vi "climbStiltLoop.vi"() -> ()   [LabVIEW 2018]
uses:
  climbStiltStateEnum.ctl
  <vilib>/Platform/TimedLoop/XDataNode/timing_clust.ctl
  <vilib>/Platform/TimedLoop/XDataNode/nitl_modes.ctl
  <vilib>/Platform/TimedLoop/XDataNode/wakeup.ctl
  <vilib>/Rock Robotics/WPI/ThirdParty/Phoenix-LabVIEW/Motor Controller/Controls/CTRE_Phoenix_MotorControl_ControlMode.ctl
  climbPlatformEnum.ctl
  <vilib>/Rock Robotics/WPI/ThirdParty/Phoenix-LabVIEW/Motor Controller/Get/CTRE_Phoenix_MotorController_GetPulseWidthAll.vi
  <vilib>/addons/control/pid/pid.llb/PID (DBL).vi
  <vilib>/platform/TimedLoop/XDataNode/XDataNode.xnode
  <vilib>/addons/control/pid/NI_PID_pid.lvlib
  <vilib>/Platform/TimedLoop/XDataNode/XDNodeRunTimeDep.lvlib
panel:
  out "Climb Stilt State LV":T1=enum."Both Retract"
  in  "Extended L2 Pos":dbl=11600.0 format="%.2f"
  in  "Crawler Wheel Power":dbl=0.8
  in  "Slow Retract Distance":dbl=1800.0 format="%#_13g"
  in  "Initial Front Retract Speed":dbl=-0.2 format="%#_13g"
  in  "Retract Output Range":cluster{"output high":dbl, "output low":dbl}={"output high"=1.0, "output low"=-1.0} {"output low" format="%.2f"; "output high" format="%.2f"}
  in  "Start Pos":dbl=1900.0 format="%.2f"
  in  "Safety Power Lower Limit":dbl=-0.1
  in  "Safety Power Upper Limit":dbl=1.0
  out "Angle Power":dbl(graph)=0.016579949830460156
  out "Pos Power":dbl(graph)=0.077
  out "Rear Power":dbl(graph)=-0.1925
  out "Front Power":dbl(graph)=-0.017
  out "Angle PID":cluster{"Angle Setpoint":dbl, dbl}(graph)={"Angle Setpoint"=0.0, -0.4144987457615042}
  out "Pos PID":cluster{"Pos Height Setpoint":dbl, dbl}(graph)={"Pos Height Setpoint"=11600.0, 11446.0}
  in  "Pos PID":T2={"proportional gain (Kc)"=0.0005, "integral time (Ti, min)"=0.0, "derivative time (Td, min)"=0.0008000000000000001} {"derivative time (Td, min)" format="%.5f"; "integral time (Ti, min)" format="%.3f"; "proportional gain (Kc)" format="%.5f"}
  in  "Angle PID":T2={"proportional gain (Kc)"=0.03999999999999997, "integral time (Ti, min)"=0.0, "derivative time (Td, min)"=0.001} {"derivative time (Td, min)" format="%.5f"; "integral time (Ti, min)" format="%.3f"; "proportional gain (Kc)" format="%.5f"}
  in  "Angle Output Range":cluster{"output high":dbl, "output low":dbl}={"output high"=0.4, "output low"=-0.4} {"output low" format="%.2f"; "output high" format="%.2f"}
  in  "Pos Output Range":cluster{"output high":dbl, "output low":dbl}={"output high"=0.85, "output low"=-0.1} {"output low" format="%.2f"; "output high" format="%.2f"}
  in  "Angle Setpoint":dbl format="%.2f"
  in  "Extended L3 Pos":dbl=27800.0 format="%.2f"
  out "Climb Angle":dbl=-0.4144987457615042
  out "Climb Pos":dbl=11446.0
  out "climbRearPosition":i32=1385
  out "climbFrontPosition":i32=1034
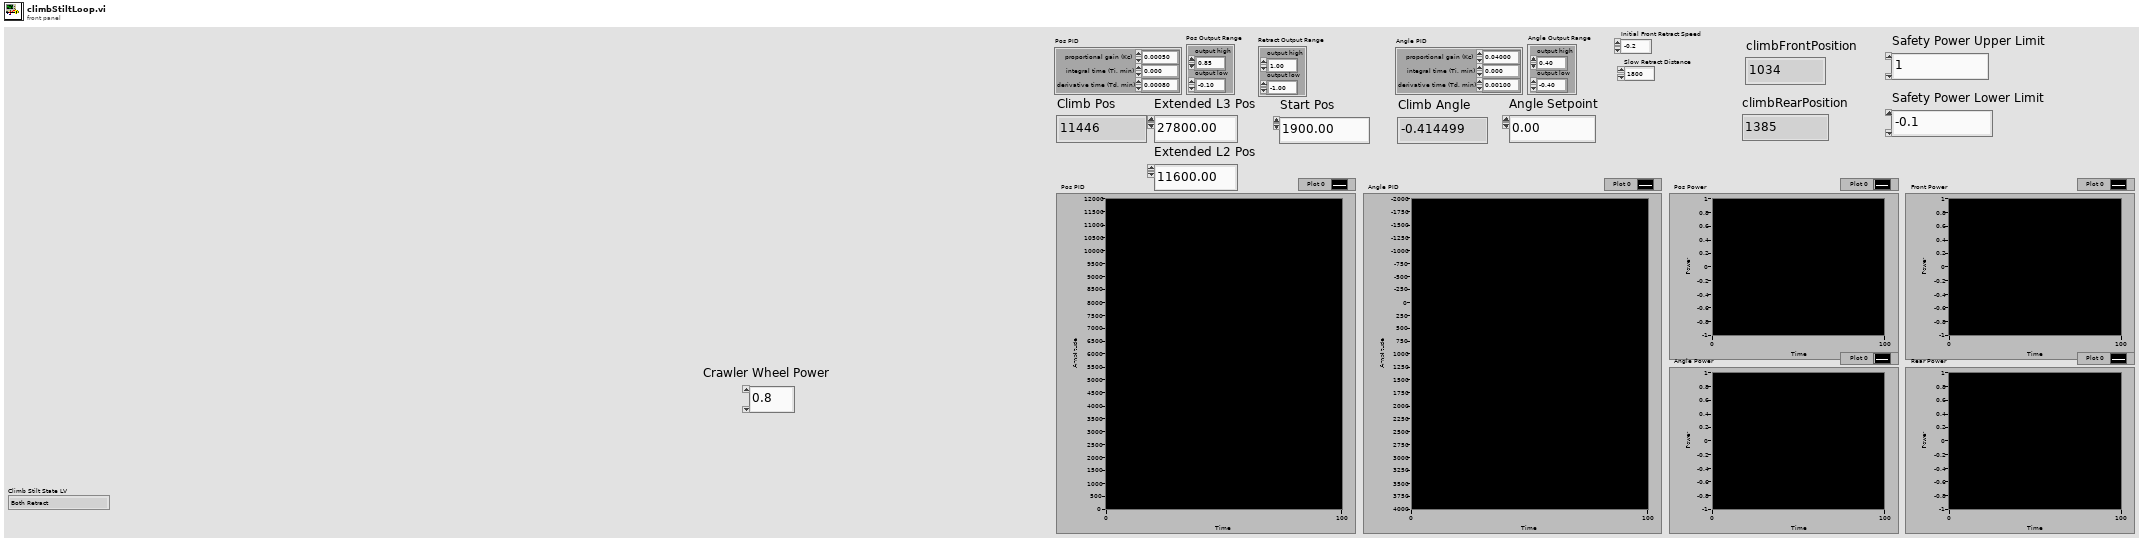
[diagram p1: front panel]
types:
  T1 = typedef "climbStiltStateEnum.ctl" = enum16{"doNothing", "Start/Safely Lower Both", "Both Extend", "Front Retract", "Both Retract"}
  T2 = cluster{"proportional gain (Kc)":dbl, "integral time (Ti, min)":dbl, "derivative time (Td, min)":dbl}
  T3 = typedef "CTRE_Phoenix_MotorControl_ControlMode.ctl" = u16
  T4 = typedef "WPI_MotorControlDeviceRef.ctl" = cluster{"DeviceStatus":errorcluster, "Type":T5, "PWM":cluster{"PWM Channel":T6, "DeadBand":T7}, "CAN":cluster{"Device Number":u8, "SetOutput VI Ref":variant, "GetOutput VI Ref":variant, "Enable VI Ref":variant, "Disable VI Ref":variant, "Data":variant}, "Invert":bool, "DIO PWM":cluster{"PWM \"Enable\" Channel":T6, "DIOChannel":T8, "PWM Rate":dbl}}
  T5 = typedef "WPI_MotorControlType.ctl" = enum16{"PWM", "CAN", "DIO PWM"}
  T6 = typedef "FPGA_DIOPWMChannel.ctl" = enum8{"PWM 0", "PWM 1", "PWM 2", "PWM 3", "PWM 4", "PWM 5", "PWM 6", "PWM 7", "PWM 8", "PWM 9", "PWM MXP 0", "PWM MXP 1", "PWM MXP 2", "PWM MXP 3", "PWM MXP 4", "PWM MXP 5", "PWM MXP 6", "PWM MXP 7", "PWM MXP 8", "PWM MXP 9", "Invalid"}
  T7 = typedef "WPI_PWMDeadband.ctl" = cluster{"Name":string, "maxPositivePwm":i32, "minPositivePwm":i32, "centerPwm":i32, "maxNegativePwm":i32, "minNegativePwm":i32, "angularRange":u16}
  T8 = typedef "FPGA_DIOChannel.ctl" = enum8{"DIO 0", "DIO 1", "DIO 2", "DIO 3", "DIO 4", "DIO 5", "DIO 6", "DIO 7", "DIO 8", "DIO 9", "DIO MXP 0", "DIO MXP 1", "DIO MXP 2", "DIO MXP 3", "DIO MXP 4", "DIO MXP 5", "DIO MXP 6", "DIO MXP 7", "DIO MXP 8", "DIO MXP 9", "DIO MXP 10", "DIO MXP 11", "DIO MXP 12", "DIO MXP 13", "DIO MXP 14", "DIO MXP 15", "SPI Port CS1", "SPI Port CS2", "SPI Port CS3", "SPI Port MISO", "SPI Port MOSI", "Invalid"}
  T9 = typedef "XDNodeRunTimeDep.lvlib/timing_clust.ctl" = cluster{"Expected End [f-1]":u64, "Actual End [f-1]":u64, "Finished Late? [f-1]":bool, "Expected End [i-1]":u64, "Actual End [i-1]":u64, "Finished Late? [i-1]":bool, "Expected Start [i]":u64, "Actual Start [i]":u64, "Expected Start [f]":u64, "Actual Start [f]":u64, "Source Name":string, "Structure Name":string, "Period":i64, "Deadline":i64, "Offset":i64, "Start":i64, "Priority":i32, "Timeout":i32, "Mode":T10, "Wakeup Reason":T11, "Error":errorcluster, "Source Type":string, "Secondary Source Type":string, "Global End Time":u64, "Global Start Time":u64, "Frame Duration":u64, "Iteration Duration":u64, "Assigned CPU":i32, "I/O Scan Engine Mode":u32}
  T10 = typedef "XDNodeRunTimeDep.lvlib/nitl_modes.ctl" = enum32{"No Change", "Process missed periods, maintain original phase", "Discard missed periods, maintain original phase", "Process missed periods, ignore original phase", "Discard missed periods, ignore original phase"}
  T11 = typedef "XDNodeRunTimeDep.lvlib/wakeup.ctl" = enum32{"Normal", "Aborted", "Asynchronous wakeup", "Timing source error", "Timed loop error", "Timeout"}
  T12 = typedef "climbPlatformEnum.ctl" = enum16{"L3 Platform", "L2 Platform"}
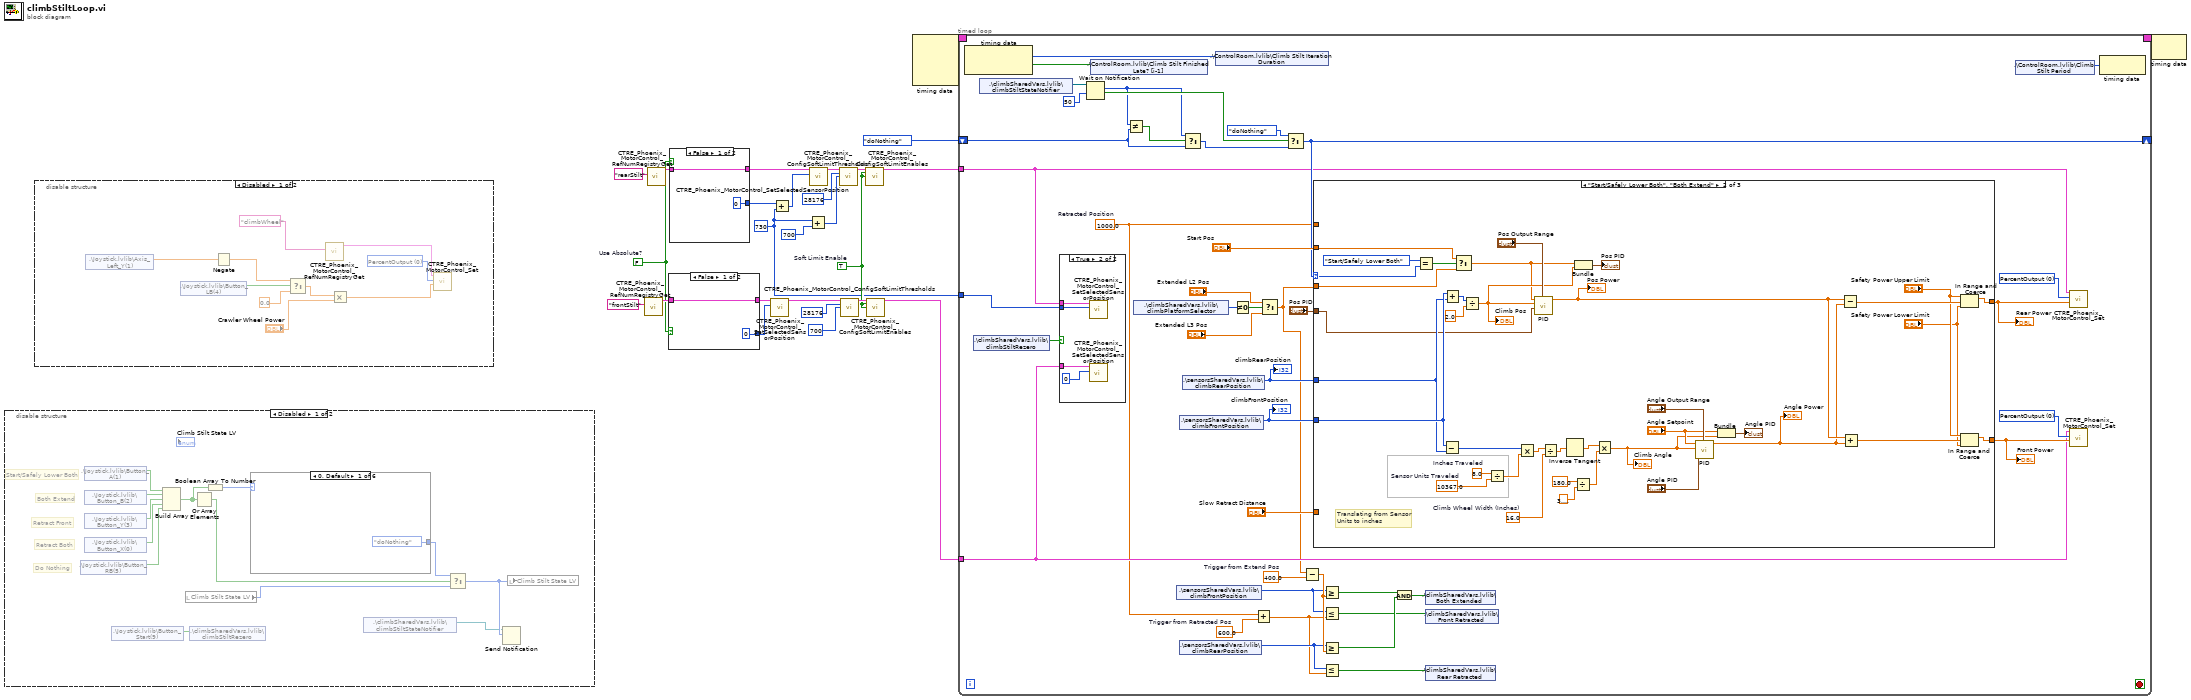
[diagram p0: block diagram]
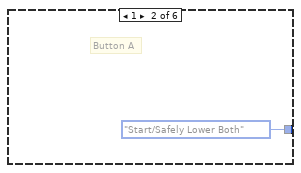
[diagram p2: hidden frame]
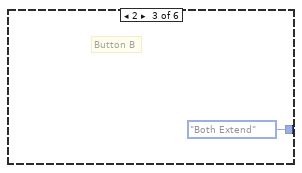
[diagram p3: hidden frame]
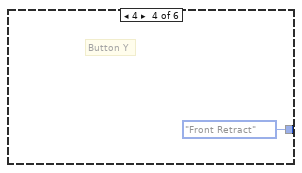
[diagram p4: hidden frame]
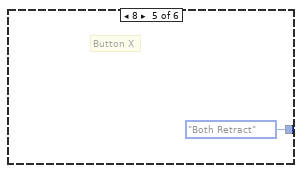
[diagram p5: hidden frame]
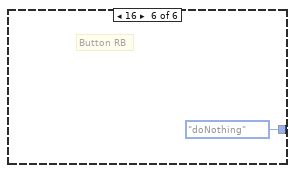
[diagram p6: hidden frame]
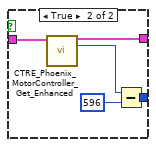
[diagram p9: hidden frame]
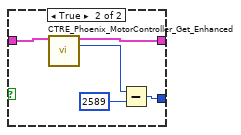
[diagram p10: hidden frame]
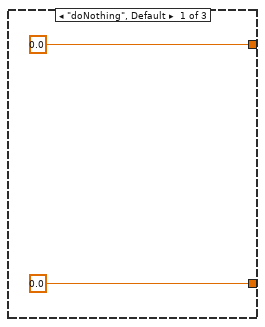
[diagram p12: hidden frame]
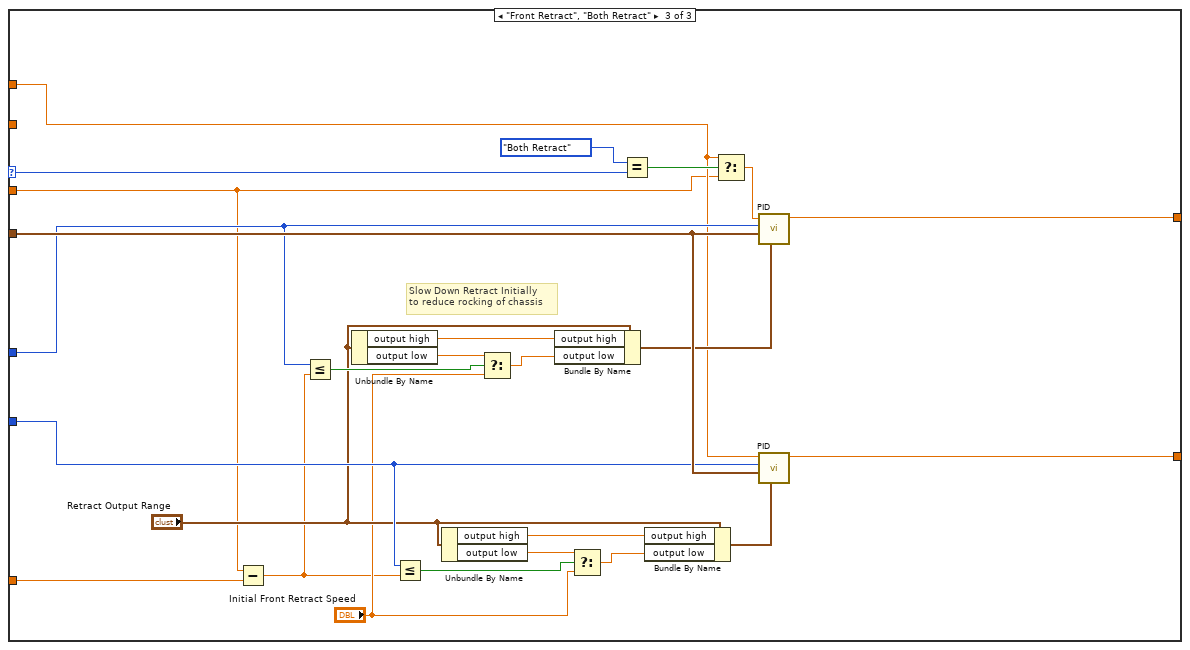
[diagram p13: hidden frame]
diagram:
  w7 = TRUE  # Soft Limit Enable
  w15 = FALSE  # Use Absolute?
  w1 = 730 ("y")
  n1 = disable-structure shown="Disabled" {
    frame Disabled {
      # "Do Nothing"
      # "Retract Both"
      # "Retract Front"
      # "Both Extend"
      # "Start/Safely Lower Both"
      n2 = shared-variable ".\\Joystick.lvlib\\Button_RB(5)"() -> (w32:bool)  [unwired: 1 in, 1 out]
      n3 = shared-variable ".\\Joystick.lvlib\\Button_A(1)"() -> (w36:bool)  [unwired: 1 in, 1 out]
      n4 = shared-variable ".\\Joystick.lvlib\\Button_B(2)"() -> (w37:bool)  [unwired: 1 in, 1 out]
      n5 = shared-variable ".\\Joystick.lvlib\\Button_Y(3)"() -> (w38:bool)  [unwired: 1 in, 1 out]
      n6 = shared-variable ".\\Joystick.lvlib\\Button_X(0)"() -> (w39:bool)  [unwired: 1 in, 1 out]
      n7 = shared-variable ".\\Joystick.lvlib\\Button_Start(9)"() -> (w27:bool)  [unwired: 1 in, 1 out]
      n8 = Build Array(w36, w37, w38, w39, w32) -> (w33:bool[])
      n9 = local read "Climb Stilt State LV"() -> (w30:T1)
      n10 = shared-variable ".\\climbSharedVars.lvlib\\climbStiltRezero"(w27) -> ()  [unwired: 1 in, 1 out]
      n11 = Or Array Elements(Boolean array=w33) -> (logical OR=w35:bool)
      n12 = Boolean Array To Number(Boolean array=w33) -> (number=w34:u32)
      n13 = case shown="0, Default" w34 {
        tunnel: [climbStiltStateEnum."doNothing" ("Climb Stilt State") climbStiltStateEnum."Start/Safely Lower Both" ("Climb Stilt State") climbStiltStateEnum."Both Extend" ("Climb Stilt State") climbStiltStateEnum."Front Retract" ("Climb Stilt State") climbStiltStateEnum."Both Retract" ("Climb Stilt State") climbStiltStateEnum."doNothing" ("Climb Stilt State")] -> w31
        frame 0, Default {
        }
        frame 1 {
          # "Button A"
        }
        frame 2 {
          # "Button B"
        }
        frame 4 {
          # "Button Y"
        }
        frame 8 {
          # "Button X"
        }
        frame 16 {
          # "Button RB"
        }
      }
      n14 = shared-variable ".\\climbSharedVars.lvlib\\climbStiltStateNotifier"() -> (w28:refnum<notifier>)  [unwired: 1 in, 1 out]
      n15 = Select(t=w31, s=w35, f=w30) -> (s? t:f=w29:T1)
      n16 = Send Notification(notification=w29, notifier=w28) -> ()  [unwired: 1 in, 2 out]
      n17 = local write "Climb Stilt State LV"(w29) -> ()
    }
    frame Enabled {
    }
  }
  n18 = disable-structure shown="Disabled" {
    frame Disabled {
      w51 = T3 0 items=["PercentOutput"=0, "Position"=1, "Velocity"=2, "Current"=3, "Follower"=5, "MotionProfile"=6, "MotionMagic"=7, "MotionProfileArc"=10, "Disabled"=15] ("Control Mode")
      n19 = shared-variable ".\\Joystick.lvlib\\Axis_Left_Y(1)"() -> (w46:dbl)  [unwired: 1 in, 1 out]
      n20 = shared-variable ".\\Joystick.lvlib\\Button_LB(4)"() -> (w55:bool)  [unwired: 1 in, 1 out]
      n21 = Negate(x=w46) -> (-x=w47:dbl)
      n22 = Select(t=w47, s=w55, f=0.0) -> (s? t:f=w53:dbl)
      n23 = call <vilib>:"CTRE_Phoenix_MotorControl_RefNumRegistryGet.vi"("refnum name"="climbWheel") -> ("PhoenixMotorControlDevRef"=w49:T4)  [unwired: 9 in, 1 out]
      n24 = Multiply(x=w53, y="Crawler Wheel Power") -> (x*y=w50:dbl)
      n25 = call <vilib>:"CTRE_Phoenix_MotorControl_Set.vi"("Output"=w50, "Control Mode"=w51, "PhoenixMotorControlDevRef"=w49) -> ()  [unwired: 7 in, 2 out]
    }
    frame Enabled {
    }
  }
  n26 = call <vilib>:"CTRE_Phoenix_MotorControl_RefNumRegistryGet.vi"("refnum name"="frontStilt") -> ("PhoenixMotorControlDevRef"=w22:T4)  [unwired: 9 in, 1 out]
  n27 = call <vilib>:"CTRE_Phoenix_MotorControl_RefNumRegistryGet.vi"("refnum name"="rearStilt") -> ("PhoenixMotorControlDevRef"=w18:T4)  [unwired: 9 in, 1 out]
  n28 = case shown="False" w15 {
    tunnel: w22 -> [w56 w62]
    tunnel: [w56 w59] -> w21
    tunnel: [0 w58] -> w20
    frame False {
    }
    frame True {
      n29 = call-poly <vilib>:"CTRE_Phoenix_MotorController_Get_Enhanced.vi"("PhoenixMotorControlDevRef"=w62) -> ("PhoenixMotorControlDevRef"=w59:T4, "Pulse Width Position"=w61:i32)  [unwired: 9 in, 4 out]
      n30 = Subtract(x=w61, y=2589) -> (x-y=w58:i32)
    }
  }
  n31 = case shown="False" w15 {
    tunnel: [0 w67] -> w19
    tunnel: w18 -> [w63 w66]
    tunnel: [w63 w65] -> w17
    frame False {
    }
    frame True {
      n32 = call-poly <vilib>:"CTRE_Phoenix_MotorController_Get_Enhanced.vi"("PhoenixMotorControlDevRef"=w66) -> ("PhoenixMotorControlDevRef"=w65:T4, "Pulse Width Position"=w68:i32)  [unwired: 9 in, 4 out]
      n33 = Subtract(x=w68, y=596) -> (x-y=w67:i32)
    }
  }
  n34 = call <vilib>:"CTRE_Phoenix_MotorControl_SetSelectedSensorPosition.vi"("New Sensor Position"=w20, "PhoenixMotorControlDevRef"=w21) -> ("PhoenixMotorControlDevRef"=w14:T4)  [unwired: 8 in, 1 out]
  n35 = Add(x=w19, y=w1) -> (x+y=w16:i32)
  n36 = call <vilib>:"CTRE_Phoenix_MotorControl_SetSelectedSensorPosition.vi"("New Sensor Position"=w16, "PhoenixMotorControlDevRef"=w17) -> ("PhoenixMotorControlDevRef"=w10:T4)  [unwired: 8 in, 1 out]
  n37 = Add(x=w1, y=700) -> (x+y=w13:i32)
  n38 = call <vilib>:"CTRE_Phoenix_MotorControl_ConfigSoftLimitThresholds.vi"("PhoenixMotorControlDevRef"=w10, "Forward Soft Limit"=28176, "Reverse Soft Limit"=w13) -> ("PhoenixMotorControlDevRef"=w9:T4)  [unwired: 11 in, 1 out]
  n39 = call <vilib>:"CTRE_Phoenix_MotorControl_ConfigSoftLimitThresholds.vi"("PhoenixMotorControlDevRef"=w14, "Forward Soft Limit"=28176, "Reverse Soft Limit"=700) -> ("PhoenixMotorControlDevRef"=w8:T4)  [unwired: 11 in, 1 out]
  n40 = call <vilib>:"CTRE_Phoenix_MotorControl_ConfigSoftLimitEnables.vi"("PhoenixMotorControlDevRef"=w9, "Forward Soft Limit Enable"=w7, "Reverse Soft Limit Enable"=w7) -> ("PhoenixMotorControlDevRef"=w5:T4)  [unwired: 11 in, 1 out]
  n41 = call <vilib>:"CTRE_Phoenix_MotorControl_ConfigSoftLimitEnables.vi"("PhoenixMotorControlDevRef"=w8, "Forward Soft Limit Enable"=w7, "Reverse Soft Limit Enable"=w7) -> ("PhoenixMotorControlDevRef"=w4:T4)  [unwired: 11 in, 1 out]
  n42 = node-c288() -> (w25:T9)  [unwired: 4 in]
  n43 = timed-loop {
    timing: w25 -> [_]
    timing-out: [_] -> w24
    tunnel: w5 -> [w86]
    tunnel: w4 -> [w85]
    shift-right: [w98] -> _
    shift-left: climbStiltStateEnum."doNothing" ("x") -> [w95]
    tunnel: w1 -> [w84]
    stop <- _ stop-if-true
    w81 = 400.0  # Trigger from Extend Pos
    w75 = 600.0  # Trigger from Retracted Pos
    w77 = 1000.0  # Retracted Position
    w106 = T3 0 items=["PercentOutput"=0, "Position"=1, "Velocity"=2, "Current"=3, "Follower"=5, "MotionProfile"=6, "MotionMagic"=7, "MotionProfileArc"=10, "Disabled"=15] ("Control Mode")
    w109 = T3 0 items=["PercentOutput"=0, "Position"=1, "Velocity"=2, "Current"=3, "Follower"=5, "MotionProfile"=6, "MotionMagic"=7, "MotionProfileArc"=10, "Disabled"=15] ("Control Mode")
    n44 = node-c288() -> (w91:i64, w90:bool)  [unwired: 1 in]
    n45 = shared-variable ".\\climbSharedVars.lvlib\\climbStiltRezero"() -> (w83:bool)  [unwired: 1 in, 1 out]
    n46 = shared-variable ".\\climbSharedVars.lvlib\\climbStiltStateNotifier"() -> (w110:refnum<notifier>)  [unwired: 1 in, 1 out]
    n47 = case shown="True" w83 {
      tunnel: w86 -> [_ w115]
      tunnel: w85 -> [_ w114]
      tunnel: w84 -> [_ w113]
      frame False {
      }
      frame True {
        n48 = call <vilib>:"CTRE_Phoenix_MotorControl_SetSelectedSensorPosition.vi"("New Sensor Position"=w113, "PhoenixMotorControlDevRef"=w115) -> ()  [unwired: 8 in, 2 out]
        n49 = call <vilib>:"CTRE_Phoenix_MotorControl_SetSelectedSensorPosition.vi"("New Sensor Position"=0, "PhoenixMotorControlDevRef"=w114) -> ()  [unwired: 8 in, 2 out]
      }
    }
    n50 = Wait on Notification(notifier=w110, timeout in ms (-1)=50) -> (notification=w92:T1, timed out?=w97:bool)  [unwired: 2 in, 2 out]
    n51 = shared-variable ".\\ControlRoom.lvlib\\Climb Stilt Finished Late? [i-1]"(w90) -> ()  [unwired: 1 in, 1 out]
    n52 = Not Equal?(x=w92, y=w95) -> (x != y?=w93:bool)
    n53 = shared-variable ".\\climbSharedVars.lvlib\\climbPlatformSelector"() -> (w99:T12)  [unwired: 1 in, 1 out]
    n54 = shared-variable ".\\sensorsSharedVars.lvlib\\climbFrontPosition"() -> (w79:i32)  [unwired: 1 in, 1 out]
    n55 = shared-variable ".\\sensorsSharedVars.lvlib\\climbFrontPosition"() -> (w108:i32)  [unwired: 1 in, 1 out]
    "climbFrontPosition" <- w108
    n56 = shared-variable ".\\sensorsSharedVars.lvlib\\climbRearPosition"() -> (w78:i32)  [unwired: 1 in, 1 out]
    n57 = shared-variable ".\\sensorsSharedVars.lvlib\\climbRearPosition"() -> (w107:i32)  [unwired: 1 in, 1 out]
    "climbRearPosition" <- w107
    n58 = Select(t=w92, s=w93, f=w95) -> (s? t:f=w94:T1)
    n59 = shared-variable ".\\ControlRoom.lvlib\\Climb Stilt Iteration Duration"(w91) -> ()  [unwired: 1 in, 1 out]
    n60 = Not Equal To 0?(x=w99) -> (x != 0?=w100:bool)
    n61 = Add(x=w77, y=w75) -> (x+y=w76:dbl)
    n62 = Select(t="Extended L2 Pos", s=w100, f="Extended L3 Pos") -> (s? t:f=w82:dbl)
    n63 = Select(t=climbStiltStateEnum."doNothing", s=w97, f=w94) -> (s? t:f=w98:T1)
    n64 = Subtract(x=w82, y=w81) -> (x-y=w80:dbl)
    n65 = case shown="\"Start/Safely Lower Both\", \"Both Extend\"" w98 {
      selector: w98 -> [_ w126 w175]
      tunnel: w108 -> [_ w153 w168]
      tunnel: w107 -> [_ w152 w162]
      tunnel: [0.0 w121 w179] -> w87
      tunnel: [0.0 w123 w180] -> w88
      tunnel: w82 -> [_ w129 w158]
      tunnel: "Start Pos" -> [_ w128 _]
      tunnel: "Pos PID" -> [_ w124 w177]
      tunnel: w77 -> [_ _ w159]
      tunnel: "Slow Retract Distance" -> [_ _ w156]
      frame "doNothing", Default {
      }
      frame "Start/Safely Lower Both", "Both Extend" {
        w136 = 10367.0  # Sensor Units Traveled
        w137 = 8.0  # Inches Traveled
        w141 = 16.0  # Climb Wheel Width (Inches)
        # "Translating from Sensor\nUnits to inches"
        n66 = Equal?(x=climbStiltStateEnum."Start/Safely Lower Both", y=w126) -> (x = y?=w127:bool)
        n67 = Subtract(x=w153, y=w152) -> (x-y=w139:i32)
        n68 = Add(x=w153, y=w152) -> (x+y=w155:i32)
        n69 = Select(t=w128, s=w127, f=w129) -> (s? t:f=w130:dbl)
        n70 = Divide(x=w155, y=2.0) -> (x/y=w148:dbl)
        "Climb Pos" <- w148
        n71 = Divide(x=w137, y=w136) -> (x/y=w138:dbl)
        n72 = Multiply(x=w139, y=w138) -> (x*y=w140:dbl)
        n73 = call-poly <vilib>:"PID.vi"("output range"="Pos Output Range", "PID gains"=w124, "process variable"=w148, "setpoint"=w130) -> ("output"=w144:dbl)  [unwired: 6 in, 1 out]
        "Pos Power" <- w144
        n74 = Divide(x=w140, y=w141) -> (x/y=w142:dbl)
        n75 = Inverse Tangent(1:w142) -> (0:w134:dbl)
        n76 = Divide(x=180.0, y=3.141592653589793) -> (x/y=w133:dbl)
        n77 = Bundle("Extended L3 Pos"=w130, w148) -> (→"Pos PID":cluster{"Extended L3 Pos":dbl, dbl})  [unwired: 1 in]
        n78 = Multiply(x=w134, y=w133) -> (x*y=w135:dbl)
        "Climb Angle" <- w135
        n79 = call-poly <vilib>:"PID.vi"("output range"="Angle Output Range", "PID gains"="Angle PID", "process variable"=w135, "setpoint"="Angle Setpoint") -> ("output"=w143:dbl)  [unwired: 6 in, 1 out]
        "Angle Power" <- w143
        n80 = Bundle("Angle Setpoint"="Angle Setpoint", w135) -> (→"Angle PID":cluster{"Angle Setpoint":dbl, dbl})  [unwired: 1 in]
        n81 = Subtract(x=w144, y=w143) -> (x-y=w122:dbl)
        n82 = Add(x=w144, y=w143) -> (x+y=w120:dbl)
        n83 = In Range and Coerce(upper limit="Safety Power Upper Limit", x=w122, lower limit="Safety Power Lower Limit") -> (coerced(x)=w123:dbl)  [unwired: 1 out]
        n84 = In Range and Coerce(upper limit="Safety Power Upper Limit", x=w120, lower limit="Safety Power Lower Limit") -> (coerced(x)=w121:dbl)  [unwired: 1 out]
      }
      frame "Front Retract", "Both Retract" {
        # "Slow Down Retract Initially\nto reduce rocking of chassis"
        n85 = Subtract(x=w158, y=w156) -> (x-y=w157:dbl)
        n86 = Less Or Equal?(x=w162, y=w157) -> (x <= y?=w164:bool)
        n87 = Unbundle By Name("Retract Output Range") -> ("output high"=w167:dbl, "output low"=w166:dbl)
        n88 = Less Or Equal?(x=w168, y=w157) -> (x <= y?=w169:bool)
        n89 = Unbundle By Name("Retract Output Range") -> ("output high"=w172:dbl, "output low"=w171:dbl)
        n90 = Select(t=w166, s=w164, f="Initial Front Retract Speed") -> (s? t:f=w165:dbl)
        n91 = Bundle By Name(cluster="Retract Output Range", "output high"=w167, "output low"=w165) -> (w160:cluster{"output high":dbl, "output low":dbl})
        n92 = Select(t=w171, s=w169, f="Initial Front Retract Speed") -> (s? t:f=w170:dbl)
        n93 = Equal?(x=climbStiltStateEnum."Both Retract", y=w175) -> (x = y?=w176:bool)
        n94 = Bundle By Name(cluster="Retract Output Range", "output high"=w172, "output low"=w170) -> (w173:cluster{"output high":dbl, "output low":dbl})
        n95 = Select(t=w159, s=w176, f=w158) -> (s? t:f=w178:dbl)
        n96 = call-poly <vilib>:"PID.vi"("output range"=w160, "PID gains"=w177, "process variable"=w162, "setpoint"=w178) -> ("output"=w180:dbl)  [unwired: 6 in, 1 out]
        n97 = call-poly <vilib>:"PID.vi"("output range"=w173, "PID gains"=w177, "process variable"=w168, "setpoint"=w159) -> ("output"=w179:dbl)  [unwired: 6 in, 1 out]
      }
    }
    "Front Power" <- w87
    "Rear Power" <- w88
    n98 = Greater Or Equal?(x=w79, y=w80) -> (x >= y?=w74:bool)
    n99 = Less Or Equal?(x=w79, y=w76) -> (x <= y?=w71:bool)
    n100 = Greater Or Equal?(x=w78, y=w80) -> (x >= y?=w73:bool)
    n101 = Less Or Equal?(x=w78, y=w76) -> (x <= y?=w70:bool)
    n102 = And(x=w74, y=w73) -> (x .and. y?=w72:bool)
    n103 = shared-variable ".\\climbSharedVars.lvlib\\Both Extended"(w72) -> ()  [unwired: 1 in, 1 out]
    n104 = shared-variable ".\\climbSharedVars.lvlib\\Front Retracted"(w71) -> ()  [unwired: 1 in, 1 out]
    n105 = shared-variable ".\\climbSharedVars.lvlib\\Rear Retracted"(w70) -> ()  [unwired: 1 in, 1 out]
    n106 = shared-variable ".\\ControlRoom.lvlib\\Climb Stilt Period"() -> (w89:i64)  [unwired: 1 in, 1 out]
    n107 = call <vilib>:"CTRE_Phoenix_MotorControl_Set.vi"("Output"=w88, "Control Mode"=w106, "PhoenixMotorControlDevRef"=w86) -> ()  [unwired: 7 in, 2 out]
    n108 = call <vilib>:"CTRE_Phoenix_MotorControl_Set.vi"("Output"=w87, "Control Mode"=w109, "PhoenixMotorControlDevRef"=w85) -> ()  [unwired: 7 in, 2 out]
    n109 = node-c288(w89) -> ()  [unwired: 1 out]
  }
  n110 = node-c288(w24) -> ()  [unwired: 1 out]
